vi "Getting Started (RX on FPGA).vi"() -> ()   [LabVIEW 2017, in "My Network Host v1.lvlib"]
uses:
  My Network Host v1.lvlib
  <vilib>/userdefined/Silver/nirio_resource_slv.ctl
  <instrlib>/_niInstr/FIFO Register Bus/v1/Host/niInstr FIFO Register Bus v1 Host.lvclass
  C:/Program Files (x86)/National Instruments/LabVIEW 2017/instr.lib/_niInstr/Instruction Framework/v1/Host/Instruction Target/niInstr Instruction Target v1 Host.lvclass
  <vilib>/FPGAPlugInAG/Dynamic/niLvFpga_Close_Dynamic.vi
  <vilib>/rvi/interface/nirviCloseFPGA/nirviCloseFPGA.xnode
  <instrlib>/_niInstr/Instruction Framework/v1/Host/Subsystem Map/niInstr Subsystem Map v1 Host.lvclass
  <instrlib>/_niInstr/Network/API/v1/Host/niInstr Network API Host v1.lvclass
panel:
  in  "UDP Destination Port":u16=35311
  in  "Stop":bool
  out "Data":u8[](array[numeric]) format="%02x"
  out "RX Waveform":u8[](graph)
  out "CLIP state":T1
  out "error out":errorcluster
  in  "resource name":T2="RIO0"
  in  "MAC Source Address":u64=1108152157446 format="%012x"
  in  "Local IP Address":string="169.254.122.138"
  in  "RX Port":i32
  # "Example Setup\nNote: Compile the \"TenGbE_Project\" FPGA Target before running this VI. Error 7 \"File not found\" most likely means the bitfile has not been compiled yet.\n\n1. Choose the resource name for your device\n2. Plug a SFP+ Direct Attach cable to the RX Port and to the transmitting Ethernet port\n3. Choose a MAC Source Address for your port.  This needs to be a unique number on the network this is attached to, and is the MAC address for the FPGA network interface\n4. Determine a unique Local IP Address for the FPGA\n5. Run this VI \n6. Run a program capable of sending data to the specified UDP Destination Port/Local IP Address"
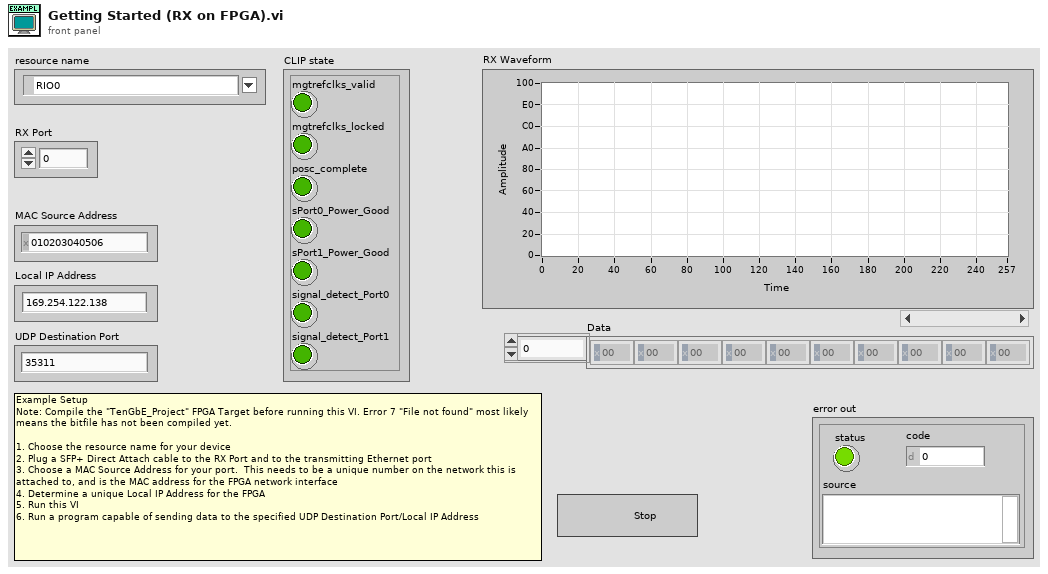
[diagram p1: front panel]
types:
  T1 = cluster{"mgtrefclks_valid":bool, "mgtrefclks_locked":bool, "posc_complete":bool, "sPort0_Power_Good":bool, "sPort1_Power_Good":bool, "signal_detect_Port0":bool, "signal_detect_Port1":bool}
  T2 = typedef "nirio_resource_slv.ctl" = tag
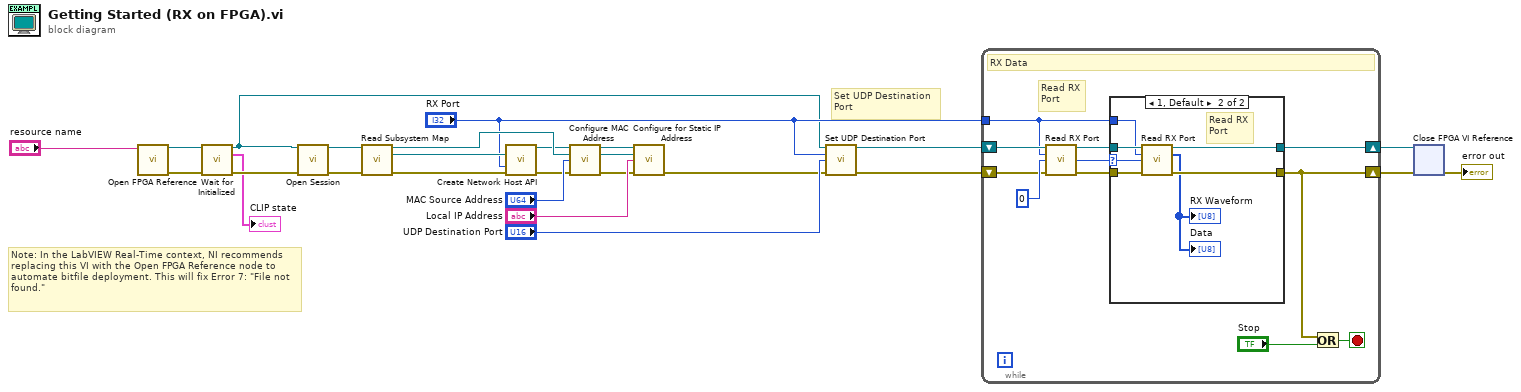
[diagram p0: block diagram]
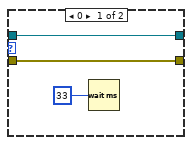
[diagram p2: hidden frame]
diagram:
  # "Set UDP Destination\nPort"
  # "Note: In the LabVIEW Real-Time context, NI recommends replacing this VI with the Open FPGA Reference node to automate bitfile deployment. This will fix Error 7: \"File not found.\""
  n1 = call "Open FPGA Reference.vi"("resource name"="resource name") -> ("FPGA VI Reference Out"=w15:refnum<k20>, "error out"=w19:errorcluster)  [unwired: 13 in]
  n2 = call "Wait for Initialized.vi"("Refnum in"=w15, "error in (no error)"=w19) -> ("Refnum out"=w1:refnum<k20>, "CLIP state"=→"CLIP state":T1, "error out"=w18:errorcluster)  [unwired: 11 in]
  n3 = call <instrlib>:"Open Session.vi"("fpga ref"=w1, "error in"=w18) -> ("session out"=w26:refnum<class "niInstr FIFO Register Bus v1 Host.lvclass">, "error out"=w22:errorcluster)  [unwired: 12 in]
  n4 = call <instrlib>:"Read Subsystem Map.vi"("instruction target in"=w26, "error in"=w22) -> ("instruction target out"=w21:refnum<class "niInstr FIFO Register Bus v1 Host.lvclass">, "subsystem map"=w25:refnum<class "niInstr Subsystem Map v1 Host.lvclass">, "error out"=w2:errorcluster)  [unwired: 11 in]
  n5 = call <instrlib>:"Create Network Host API.vi"("subsystem map"=w25, "instance number"="RX Port", "error in (no error)"=w2) -> ("niInstr Network API Host v1 out"=w16:refnum<class "niInstr Network API Host v1.lvclass">, "error out"=w17:errorcluster)  [unwired: 11 in]
  n6 = call <instrlib>:"Configure MAC Address.vi"("niInstr Network API Host v1 in"=w16, "instruction target in"=w21, "Local MAC Address"="MAC Source Address", "error in (no error)"=w17) -> ("niInstr Network API Host v1 out"=w6:refnum<class "niInstr Network API Host v1.lvclass">, "instruction target out"=w4:refnum<class "niInstr FIFO Register Bus v1 Host.lvclass">, "error out"=w5:errorcluster)  [unwired: 9 in]
  n7 = call <instrlib>:"Configure for Static IP Address.vi"("niInstr Network API Host v1 in"=w6, "instruction target in"=w4, "Local IP Address"="Local IP Address", "error in (no error)"=w5) -> ("error out"=w7:errorcluster)  [unwired: 9 in, 2 out]
  n8 = call "Set UDP Destination Port.vi"("Refnum in"=w1, "ethernet port"="RX Port", "UDP Destination Port"="UDP Destination Port", "error in (no error)"=w7) -> ("Refnum out"=w11:refnum<k20>, "error out"=w12:errorcluster)  [unwired: 10 in]
  n9 = while {
    shift-right: [w36] -> w9
    shift-left: w12 -> [w30]
    shift-right: [w29] -> w10
    shift-left: w11 -> [w28]
    tunnel: "RX Port" -> [w27]
    stop <- w37 stop-if-true
    # "Read RX\nPort"
    # "RX Data"
    n10 = call "Read RX Port.vi"("Refnum in"=w28, "Ethernet port"=w27, "Elements to Read"=u32 0 ("Number of Elements"), "error in (no error)"=w30) -> ("Refnum out"=w34:refnum<k20>, "Elements Remaining out"=w32:u32, "error out"=w33:errorcluster)  [unwired: 8 in, 1 out]
    n11 = case shown="1, Default" w32 {
      selector: w32 -> [_ w42]
      tunnel: w34 -> [w38 w47]
      tunnel: w33 -> [w39 w46]
      tunnel: [w39 w45] -> w36
      tunnel: [w38 w43] -> w29
      tunnel: w27 -> [_ w41]
      frame 0 {
        n12 = Wait (ms)(milliseconds to wait=u32 33) -> ()  [unwired: 1 out]
      }
      frame 1, Default {
        # "Read RX\nPort"
        n13 = call "Read RX Port.vi"("Refnum in"=w47, "Ethernet port"=w41, "Elements to Read"=w42, "error in (no error)"=w46) -> ("Refnum out"=w43:refnum<k20>, "Data"=→"Data" →"RX Waveform":u8[], "error out"=w45:errorcluster)  [unwired: 8 in, 1 out]
      }
    }
    n14 = Or(x=w36, y="Stop") -> (x .or. y?=w37:bool)
  }
  n15 = xnode "Close FPGA VI Reference"("FPGA VI Reference In"=w10, "error in"=w9) -> ("error out"=→"error out":errorcluster)
